vi "N DBL to Result.vi"(8 "error in (no error)":errorcluster, 9 "Data":dbl[](array[numeric]), 10 "Result in":refnum<class "Acquired Result.lvclass">, 11 "Instrument Driver in":refnum<class "Instrument Driver.lvclass">) -> (0 "error out":errorcluster, 2 "Result out":refnum<class "Acquired Result.lvclass">, 3 "Instrument Driver out":refnum<class "Instrument Driver.lvclass">)   [LabVIEW 2016, in "Instrument Driver.lvclass"]
uses:
  Instrument Driver.lvclass
  Results/Acquired Result/Acquired Result.lvclass
  Instrument Driver.lvclass/Instrument Driver.ctl
  Results/Acquired Result/Acquired Result.lvclass/Acquired Result.ctl
  Read Channel names.vi
  Read Group name.vi
  Read Channel units.vi
  Read Timing group name.vi
  Results/Acquired Result/Write Channels.vi
  Results/Acquired Result/Write Group.vi
  Results/Acquired Result/Write Time group.vi
  Results/Acquired Result/Write Time value.vi
  <vilib>/express/express shared/transition.llb/Dynamic To Waveform Array.vi
  <vilib>/express/express signal manip/GetorSetDDTAttributes/Set DDT Attributes/SetT0.vi
  <vilib>/express/express shared/transition.llb/Waveform Array To Dynamic.vi
  <vilib>/express/express signal manip/GetorSetDDTAttributes/Set DDT Attributes/Set DDT Properties.xnode
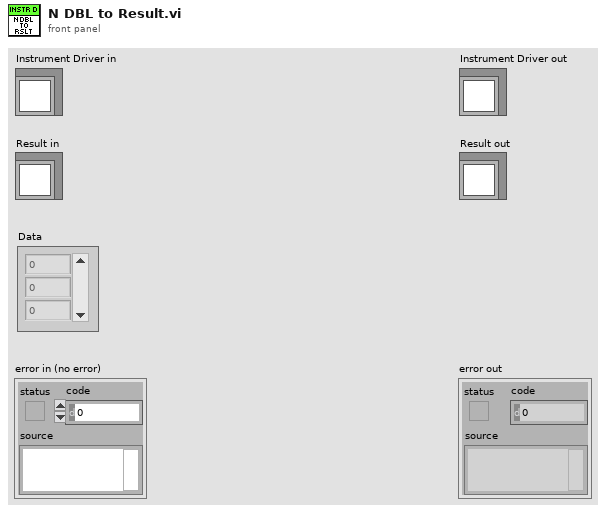
[diagram p1: front panel]
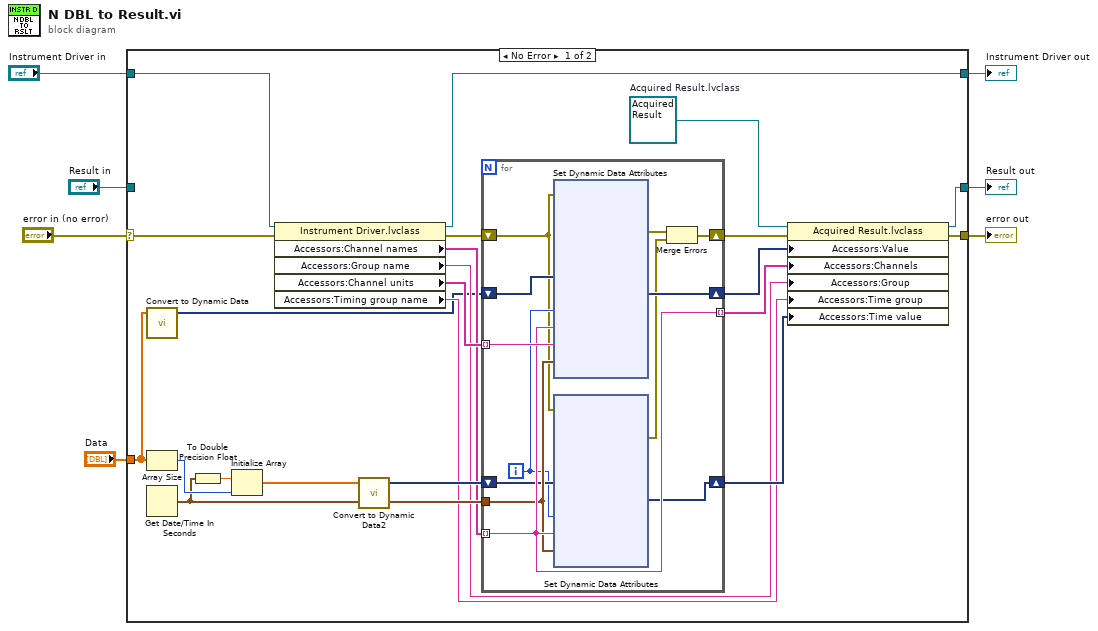
[diagram p0: block diagram]
diagram:
  n1 = case shown="No Error" "error in (no error)" {
    selector: "error in (no error)" -> [w13 w82]
    tunnel: [w10 w82] -> w6
    tunnel: [w8 w81] -> w4
    tunnel: "Instrument Driver in" -> [w9 w81]
    tunnel: "Data" -> [w12 _]
    tunnel: [w11 w80] -> w2
    tunnel: "Result in" -> [_ w80]
    frame No Error {
      w16 = refnum<class "Acquired Result.lvclass"> refnum  # Acquired Result.lvclass
      n2 = call "Convert to Dynamic Data"("Array"=w12) -> ("Dynamic Data Type"=w15:dynamicdata)  [unwired: 3 in]
      n3 = Array Size(array=w12) -> (size(s)=w29:i32)
      n4 = Get Date/Time In Seconds() -> (seconds since 1Jan1904=w24:timestamp)
      n5 = To Double Precision Float(number=w24) -> (double precision float=w25:dbl)
      n6 = Initialize Array(w25, w29) -> (w26:dbl[])
      n7 = property class="Instrument Driver.lvclass"(reference=w9, error in=w13) -> (reference out=w8:refnum<class "Instrument Driver.lvclass">, error out=w22:errorcluster, "Accessors:Channel names"=w19:string[], "Accessors:Group name"=w20:string, "Accessors:Channel units"=w21:string[], "Accessors:Timing group name"=w23:string)
      n8 = call "Convert to Dynamic Data2"("Array"=w26) -> ("Dynamic Data Type"=w27:dynamicdata)  [unwired: 3 in]
      n9 = for {
        tunnel: [w37] -> w18 mode=indexing
        tunnel: w19 -> [w37] mode=indexing
        tunnel: w21 -> [w38] mode=indexing
        shift-right: [w39] -> w14
        shift-left: w15 -> [w40]
        shift-right: [w31] -> w17
        shift-left: w22 -> [w32]
        tunnel: w24 -> [w36]
        shift-right: [w33] -> w28
        shift-left: w27 -> [w35]
        i -> [w34]
        n10 = xnode "Set Dynamic Data Attributes"("Signals In"=w40, "Signal Index"=w34, "Signal Name"=w37, "Unit"=w38, "Timestamp"=w36, "error in"=w32) -> ("Signals Out"=w39:dynamicdata, "error out"=w41:errorcluster)
        n11 = xnode "Set Dynamic Data Attributes"("Signals In"=w35, "Signal Index"=w34, "Signal Name"=w37, "Timestamp"=w36, "error in"=w32) -> ("Signals Out"=w33:dynamicdata, "error out"=w30:errorcluster)
        n12 = Merge Errors(w41, w30) -> (w31:errorcluster)
      }
      n13 = property class="Acquired Result.lvclass"(reference=w16, error in=w17, "Accessors:Value"=w14, "Accessors:Channels"=w18, "Accessors:Group"=w20, "Accessors:Time group"=w23, "Accessors:Time value"=w28) -> (reference out=w11:refnum<class "Acquired Result.lvclass">, error out=w10:errorcluster)
    }
    frame Error {
    }
  }
  "error out" <- w6
  "Instrument Driver out" <- w4
  "Result out" <- w2
